vi "Main.vi"() -> ()   [LabVIEW 2015]
doc: "This template is for the Queued Message Handler design pattern.\n\nThe Event Handling Loop generates messages based on user interface actions.\n\nThe Message Handling Loop processes messages generated by the Event Handling Loop, or by other messages. The messages are string values, so new messages can be added easily to the Message Cases case structure in the Message Handling Loop. Each message cluster can also provide an optional value for Message Data, which is a variant that can be converted to whatever message-specific data is required."
uses:
  controls/UI Data.ctl
  support/Message Queue/Message Queue.lvlib
  support/User Event - Stop/User Event - Stop.lvlib
  support/Message Queue/Enqueue Message (Single).vi
  <vilib>/ErrorRing/Error Ring.xnode
  PL Model/PL Model.lvlib
  DAQ/DAQ.lvlib
  DAQ/TypeDefs/DAQ data.ctl
  support/Exit Notifiers/PLC Notifiers.lvlib
  <vilib>/Utility/error.llb/Error Cluster From Error Code.vi
  Logger/Logger.lvlib
  support/Status Logger/Status Log.ctl
panel:
  in  "Abort":bool
  in  "Stop Line":bool
  in  "Start Line":bool
  out "Status":string
  in  "Tab Control":enum32{"DAQ simulation", "DAQ control"}(tab)
  in  "Positon":dbl(slide) scale=0.0..20.0
  in  "Dispose":bool
  in  "Pump":bool
  in  "Flow [l/s]":dbl=10.0
  in  "Position (AI potentiometer)":tag
  in  "Pump (DO LED)":tag
  in  "Main switch (DI bistable switch)":tag
  in  "Dispose barrel (DI monostable switch)":tag
  in  "Exit":bool
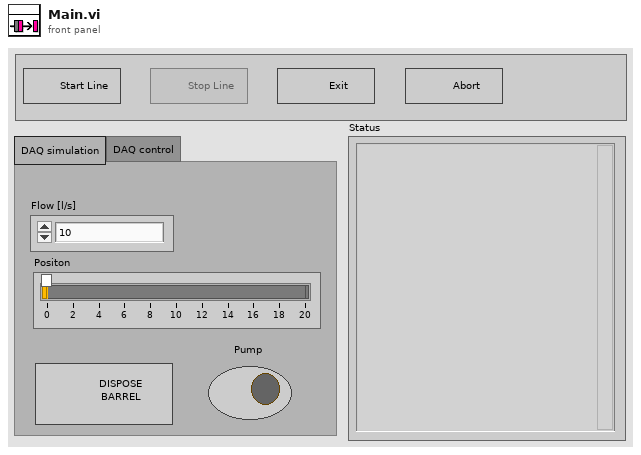
[diagram p1: front panel]
types:
  T1 = typedef "Status Log.ctl" = enum16{"Close file", "Open Status file", "Add Status", "Get file path"}
  T2 = typedef "UI Data.ctl" = cluster{"Status":string, "Start Line Ref":refnum<vi>, "Stop Line Ref":refnum<vi>, "Data Display Ref":refnum<vi>, "Exit Button Ref":refnum<vi>, "Pump Ref":refnum<vi>, "Dispose Ref":refnum<vi>, "Flow Ref":refnum<vi>, "Position Ref":refnum<vi>, "Tab Ref":refnum<vi>}
  T3 = typedef "PLC Notifiers.lvlib/PLC Notifiers.ctl" = cluster{"PL Model Exit":refnum<notifier>, "DAQ Exit":refnum<notifier>, "PLC Exit":refnum<notifier>}
  T4 = typedef "Message Queue.lvlib/All Message Queues.ctl" = cluster{"UI":refnum<queue>, "PL Model":refnum<queue>, "DAQ":refnum<queue>, "PLC":refnum<queue>, "Loger":refnum<queue>}
  T5 = typedef "DAQ.lvlib/DAQ data.ctl" = cluster{"Power switch (DI)":cluster{"Channel":tag, "Data":bool}, "Dispose barrel (DI)":cluster{"Channel":tag, "Data":bool}, "Pump status (DO)":cluster{"Channel":tag, "Data":bool}, "Barrel position (AI)":cluster{"Channel":tag, "Data":dbl}}
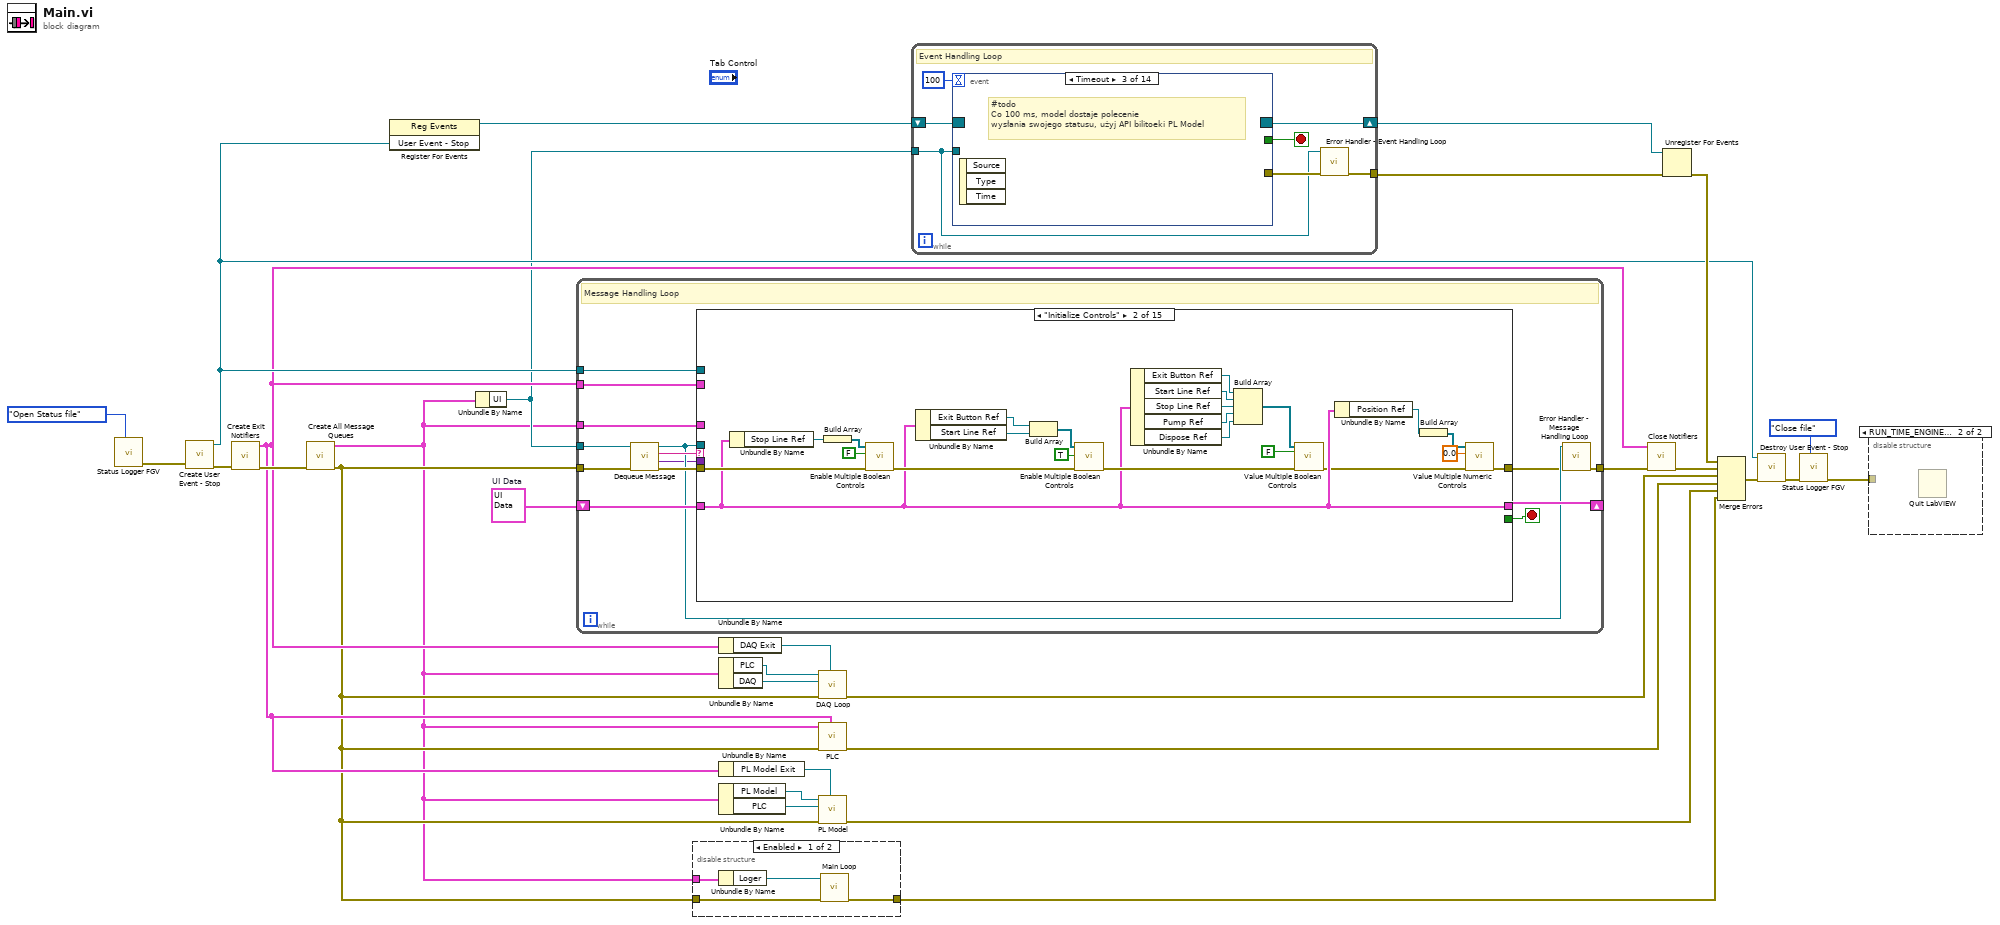
[diagram p0: block diagram]
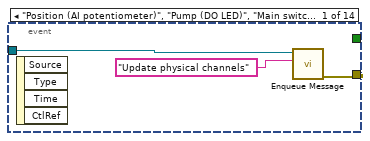
[diagram p2: hidden frame]
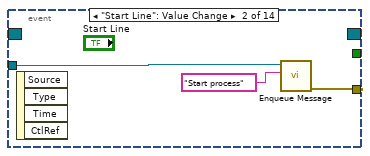
[diagram p3: hidden frame]
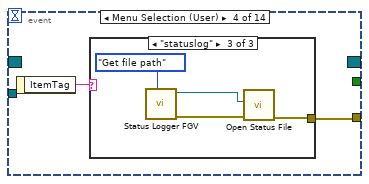
[diagram p4: hidden frame]
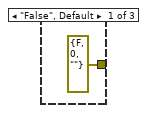
[diagram p5: hidden frame]
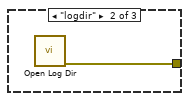
[diagram p6: hidden frame]
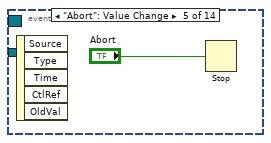
[diagram p7: hidden frame]
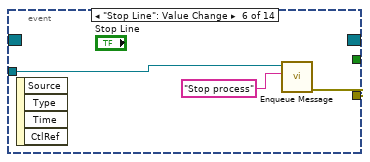
[diagram p8: hidden frame]
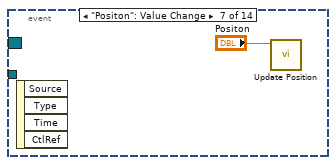
[diagram p9: hidden frame]
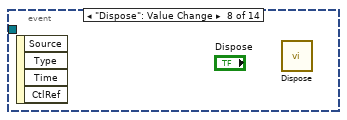
[diagram p10: hidden frame]
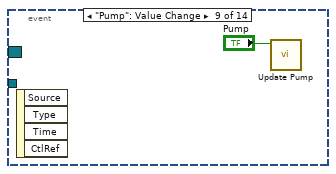
[diagram p11: hidden frame]
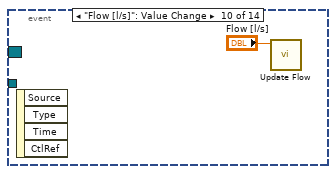
[diagram p12: hidden frame]
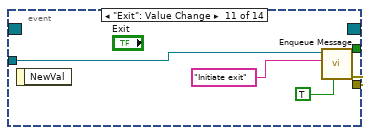
[diagram p13: hidden frame]
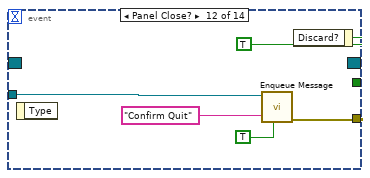
[diagram p14: hidden frame]
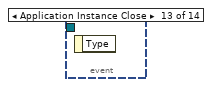
[diagram p15: hidden frame]
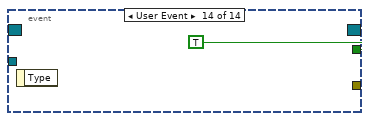
[diagram p16: hidden frame]
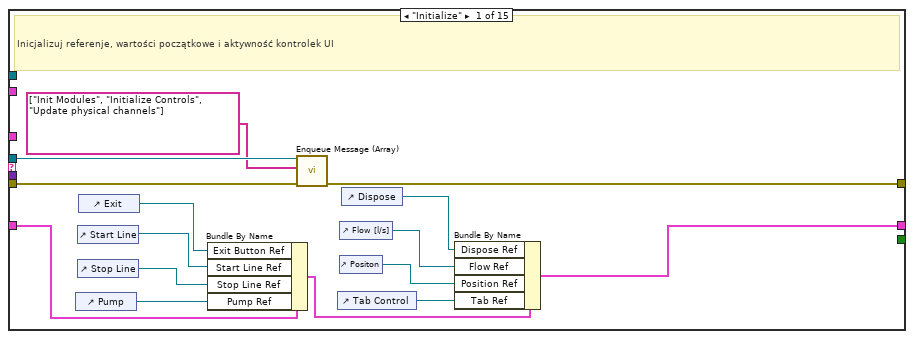
[diagram p18: hidden frame]
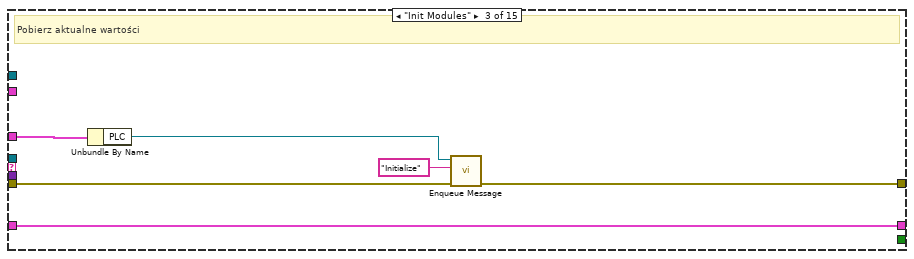
[diagram p19: hidden frame]
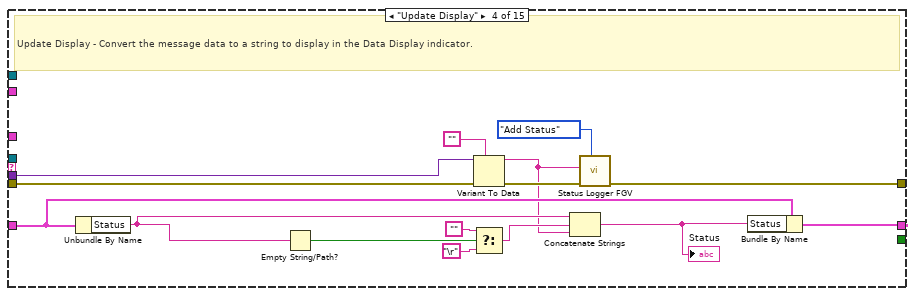
[diagram p20: hidden frame]
diagram:
  w27 = T2 {"Status"="", "Start Line Ref"=refnum, "Stop Line Ref"=refnum, "Data Display Ref"=refnum, "Exit Button Ref"=refnum, "Pump Ref"=refnum, "Dispose Ref"=refnum, "Flow Ref"=refnum, "Position Ref"=refnum, "Tab Ref"=refnum}  # UI Data
  n1 = call "Status Logger FGV.vi"("Action"=Status_Log."Open Status file") -> ("error out"=w4:errorcluster)  [unwired: 9 in, 1 out]
  n2 = call "Create User Event - Stop.vi"("error in (no error)"=w4) -> ("error out"=w19:errorcluster, "User Event - Stop"=w23:refnum<user-event>)  [unwired: 9 in]
  n3 = call "Create Exit Notifiers.vi"("error in"=w19) -> ("error out"=w18:errorcluster, "Notifiers"=w15:T3)  [unwired: 9 in]
  n4 = call "Create All Message Queues.vi"("error in (no error)"=w18) -> ("error out"=w9:errorcluster, "Message Queues out"=w7:T4)  [unwired: 9 in]
  n5 = register-events(w23) -> (reference out=w24:refnum<event-registration>)  [unwired: 2 in, 1 out]
  n6 = Unbundle By Name(w7) -> ("UI"=w8:refnum<queue>)
  n7 = while {
    tunnel: w8 -> [w37]
    shift-right: [w43] -> _
    shift-left: w27 -> [w44]
    tunnel: w23 -> [w41]
    tunnel: w9 -> [w40]
    tunnel: [w35] -> w17
    tunnel: w7 -> [w33]
    tunnel: w15 -> [w32]
    stop <- w42 stop-if-true
    # "Message Handling Loop"
    n8 = call "Dequeue Message.vi"("error in (no error)"=w40, "Message Queue"=w37) -> ("error out"=w39:errorcluster, "Message Data"=w31:variant, "Message"=w38:string, "dup Message Queue"=w36:refnum<queue>)  [unwired: 6 in]
    n9 = case "Message Cases" shown="\"Initialize Controls\"" w38 {
      selector: w38 -> [_ _ _ _ _ _ _ _ _ _ _ _ _ w226 _]
      tunnel: w36 -> [w56 _ _ _ _ _ w149 w159 _ w181 w191 w218 _ _ _]
      tunnel: w39 -> [w57 w82 w85 w103 w110 w119 w152 w163 w174 w177 w193 w209 w225 _ w238]
      tunnel: [w58 w63 w87 w89 w116 w136 w154 w161 w172 w188 w190 w207 w219 w227 w236] -> w34
      tunnel: w44 -> [w59 w65 w84 w99 w117 w125 w141 w162 w170 w189 w197 w217 w224 w228 w237]
      tunnel: [w47 w65 w84 w97 w117 w125 w141 w162 w170 w189 w197 w217 w224 w228 w237] -> w43
      tunnel: [_ _ _ _ _ _ _ _ _ _ _ TRUE _ _ _] -> w42
      tunnel: w31 -> [_ _ _ w102 _ _ _ _ w173 _ _ w210 w223 _ _]
      tunnel: w41 -> [_ _ _ _ _ _ _ _ _ _ _ w214 _ _ _]
      tunnel: w33 -> [_ _ w83 _ w106 w135 w153 _ _ w187 _ _ _ _ _]
      tunnel: w32 -> [_ _ _ _ _ _ _ _ _ _ w196 _ _ _ _]
      frame "Initialize" {
        # "Inicjalizuj referenje, wartości początkowe i aktywność kontrolek UI"
        n10 = control-ref of="Pump"() -> (w51:refnum<vi>)
        n11 = control-ref of="Start Line"() -> (w53:refnum<vi>)
        n12 = control-ref of="Stop Line"() -> (w52:refnum<vi>)
        n13 = control-ref of="Exit"() -> (w54:refnum<vi>)
        n14 = Bundle By Name(cluster=w59, "Exit Button Ref"=w54, "Start Line Ref"=w53, "Stop Line Ref"=w52, "Pump Ref"=w51) -> (w55:T2)
        n15 = call "Enqueue Message (Array).vi"("error in (no error)"=w57, "Message Array"=string[] ["Init Modules", "Initialize Controls", "Update physical channels"], "Message Queue"=w56) -> ("error out"=w58:errorcluster)  [unwired: 7 in, 1 out]
        n16 = control-ref of="Tab Control"() -> (w50:refnum<vi>)
        n17 = control-ref of="Flow [l/s]"() -> (w48:refnum<vi>)
        n18 = control-ref of="Positon"() -> (w49:refnum<vi>)
        n19 = control-ref of="Dispose"() -> (w46:refnum<vi>)
        n20 = Bundle By Name(cluster=w55, "Dispose Ref"=w46, "Flow Ref"=w48, "Position Ref"=w49, "Tab Ref"=w50) -> (w47:T2)
      }
      frame "Initialize Controls" {
        n21 = Unbundle By Name(w65) -> ("Stop Line Ref"=w80:refnum<vi>)
        n22 = Build Array(w80) -> (w79:refnum<vi>[])
        n23 = call "Enable Multiple Boolean Controls.vi"("error in (no error)"=w82, "Enabled"=FALSE, "References"=w79) -> ("error out"=w76:errorcluster)  [unwired: 8 in]
        n24 = Unbundle By Name(w65) -> ("Exit Button Ref"=w78:refnum<vi>, "Start Line Ref"=w77:refnum<vi>)
        n25 = Build Array(w78, w77) -> (w75:refnum<vi>[])
        n26 = call "Enable Multiple Boolean Controls.vi"("error in (no error)"=w76, "Enabled"=TRUE, "References"=w75) -> ("error out"=w68:errorcluster)  [unwired: 8 in]
        n27 = Unbundle By Name(w65) -> ("Exit Button Ref"=w73:refnum<vi>, "Start Line Ref"=w72:refnum<vi>, "Stop Line Ref"=w71:refnum<vi>, "Pump Ref"=w70:refnum<vi>, "Dispose Ref"=w69:refnum<vi>)
        n28 = Build Array(w73, w72, w71, w70, w69) -> (w66:refnum<vi>[])
        n29 = call "Value Multiple Boolean Controls.vi"("error in (no error)"=w68, "Enabled"=FALSE, "References"=w66) -> ("error out"=w64:errorcluster)  [unwired: 8 in]
        n30 = Unbundle By Name(w65) -> ("Position Ref"=w62:refnum<vi>)
        n31 = Build Array(w62) -> (w61:refnum<vi>[])
        n32 = call "Value Multiple Numeric Controls.vi"("error in (no error)"=w64, "Value"=0.0, "References"=w61) -> ("error out"=w63:errorcluster)  [unwired: 8 in]
      }
      frame "Init Modules" {
        # "Pobierz aktualne wartości"
        n33 = Unbundle By Name(w83) -> ("PLC"=w86:refnum<queue>)
        n34 = call-poly "Enqueue Message.vi"("error in (no error)"=w85, "Message"="Initialize", "Message Queue"=w86) -> ("error out"=w87:errorcluster)  [unwired: 7 in, 1 out]
      }
      frame "Update Display" {
        # "Update Display - Convert the message data to a string to display in the Data Display indicator."
        n35 = Unbundle By Name(w99) -> ("Status"=w96:string)
        n36 = Empty String/Path?(string/path=w96) -> (empty?=w95:bool)
        n37 = Variant To Data(error in=w103, type="", Variant=w102) -> (data=w91:string, error out=w100:errorcluster)
        n38 = Select(t="", s=w95, f="\r") -> (s? t:f=w92:string)
        n39 = Concatenate Strings(w96, w92, w91) -> (w98:string)
        "Status" <- w98
        n40 = call "Status Logger FGV.vi"("Action"=Status_Log."Add Status", "error in (no error)"=w100, "Status"=w91) -> ("error out"=w89:errorcluster)  [unwired: 7 in, 1 out]
        n41 = Bundle By Name(cluster=w99, "Status"=w98) -> (w97:T2)
      }
      frame "Update physical channels" {
        # "Duplicate this frame when creating new messages.  Change this comment in the duplicated frame to describe this message."
        n42 = Bundle By Name(cluster=T5 {"Power switch (DI)"={"Channel"="", "Data"=FALSE}, "Dispose barrel (DI)"={"Channel"="", "Data"=FALSE}, "Pump status (DO)"={"Channel"="", "Data"=FALSE}, "Barrel position (AI)"={"Channel"="", "Data"=0.0}} ("DAQ data"), "Power switch (DI).Channel"="Main switch (DI bistable switch)", "Pump status (DO).Channel"="Pump (DO LED)", "Barrel position (AI).Channel"="Position (AI potentiometer)", "Dispose barrel (DI).Channel"="Dispose barrel (DI monostable switch)") -> (w108:T5)
        n43 = Unbundle By Name(w106) -> ("PLC"=w105:refnum<queue>)
        n44 = To Variant(anything=w108) -> (Variant=w107:variant)
        n45 = call-poly "Enqueue Message.vi"("error in (no error)"=w110, "Message Data"=w107, "Message"="Update channels", "Message Queue"=w105) -> ("error out"=w109:errorcluster)  [unwired: 6 in, 1 out]
        n46 = Merge Errors(w109) -> (w116:errorcluster)
      }
      frame "Start process" {
        # "Duplicate this frame when creating new messages.  Change this comment in the duplicated frame to describe this message."
        n47 = Unbundle By Name(w125) -> ("Start Line Ref"=w128:refnum<vi>)
        n48 = Unbundle By Name(w125) -> ("Stop Line Ref"=w124:refnum<vi>)
        n49 = Unbundle By Name(w135) -> ("UI"=w121:refnum<queue>, "PLC"=w134:refnum<queue>, "Loger"=w118:refnum<queue>)
        n50 = call "Open Log.vi"("error in (no error)"=w119, "Message Queue"=w118) -> ("error out"=w120:errorcluster)  [unwired: 9 in]
        n51 = Build Array(w128) -> (w127:refnum<vi>[])
        n52 = Build Array(w124) -> (w123:refnum<vi>[])
        n53 = call-poly "Enqueue Message.vi"("error in (no error)"=w120, "Message"="Start", "Message Queue"=w134) -> ("error out"=w132:errorcluster)  [unwired: 7 in, 1 out]
        n54 = call "Enable Multiple Boolean Controls.vi"("Enabled"=FALSE, "References"=w127) -> ()  [unwired: 9 in, 1 out]
        n55 = call "Enable Multiple Boolean Controls.vi"("Enabled"=TRUE, "References"=w123) -> ()  [unwired: 9 in, 1 out]
        n56 = call-poly "Enqueue Message.vi"("error in (no error)"=w132, "Message Data"="Starting production line..." ("Message"), "Message"="Update Display", "Message Queue"=w121) -> ("error out"=w131:errorcluster)  [unwired: 6 in, 1 out]
        n57 = Merge Errors(w131) -> (w136:errorcluster)
      }
      frame "Stop process" {
        # "Duplicate this frame when creating new messages.  Change this comment in the duplicated frame to describe this message."
        n58 = Unbundle By Name(w141) -> ("Start Line Ref"=w144:refnum<vi>)
        n59 = Unbundle By Name(w141) -> ("Stop Line Ref"=w140:refnum<vi>)
        n60 = Unbundle By Name(w153) -> ("PLC"=w151:refnum<queue>)
        n61 = Build Array(w144) -> (w143:refnum<vi>[])
        n62 = Build Array(w140) -> (w139:refnum<vi>[])
        n63 = call-poly "Enqueue Message.vi"("error in (no error)"=w152, "Message"="Stop", "Message Queue"=w151) -> ("error out"=w148:errorcluster)  [unwired: 7 in, 1 out]
        n64 = To Variant(anything="Stopping production line..." ("Message")) -> (Variant=w137:variant)
        n65 = call "Enable Multiple Boolean Controls.vi"("Enabled"=TRUE, "References"=w143) -> ()  [unwired: 9 in, 1 out]
        n66 = call "Enable Multiple Boolean Controls.vi"("Enabled"=FALSE, "References"=w139) -> ()  [unwired: 9 in, 1 out]
        n67 = call-poly "Enqueue Message.vi"("error in (no error)"=w148, "Message Data"=w137, "Message"="Update Display", "Message Queue"=w149) -> ("error out"=w147:errorcluster)  [unwired: 6 in, 1 out]
        n68 = Merge Errors(w147) -> (w154:errorcluster)
      }
      frame "Confirm Quit" {
        # "Confirm Quit - Message that can confirm whether or not the user wants to exit the application."
        n69 = Two Button Dialog(message="Are you sure?", 1:"Continue" ("F button name (\"Cancel\")"), 2:"Quit" ("T button name (\"OK\")")) -> (T button?=w155:bool)
        n70 = case shown="True" w155 {
          tunnel: w163 -> [w164 w169]
          tunnel: [w164 w168] -> w160
          tunnel: w159 -> [_ w167]
          frame False {
          }
          frame True {
            n71 = call-poly "Enqueue Message.vi"("Priority Message? (F)"=TRUE, "error in (no error)"=w169, "Message"="Initiate exit", "Message Queue"=w167) -> ("error out"=w168:errorcluster)  [unwired: 6 in, 1 out]
          }
        }
        n72 = Merge Errors(w160) -> (w161:errorcluster)
      }
      frame "Update PL Status" {
        n73 = Variant To Data(error in=w174, type="", Variant=w173) -> (error out=w172:errorcluster)  [unwired: 1 out]
      }
      frame "Initiate exit" {
        # "Exit - Exit the application."
        n74 = Unbundle By Name(w187) -> ("PLC"=w186:refnum<queue>, "Loger"=w175:refnum<queue>)
        n75 = call "Exit.vi"("error in (no error)"=w177, "Message Queue"=w175) -> ("error out"=w176:errorcluster)  [unwired: 9 in]
        n76 = call-poly "Enqueue Message.vi"("Priority Message? (F)"=TRUE, "error in (no error)"=w176, "Message"="Exit PLC", "Message Queue"=w186) -> ("error out"=w179:errorcluster)  [unwired: 6 in, 1 out]
        n77 = Flush Queue(queue=w181, error in (no error)=w179) -> (queue out=w180:refnum<queue>, error out=w178:errorcluster)  [unwired: 1 out]
        n78 = call-poly "Enqueue Message.vi"("error in (no error)"=w178, "Message"="Wait on PLC exit", "Message Queue"=w180) -> ("error out"=w184:errorcluster)  [unwired: 7 in, 1 out]
        n79 = Merge Errors(w184) -> (w188:errorcluster)
      }
      frame "Wait on PLC exit" {
        # "Exit - Exit the application."
        n80 = Unbundle By Name(w196) -> ("PLC Exit"=w195:refnum<notifier>)
        n81 = Wait on Notification(notifier=w195, timeout in ms (-1)=10, error in (no error)=w193) -> (timed out?=w192:bool)  [unwired: 1 in, 3 out]
        n82 = case shown="True" w192 {
          tunnel: [w200 w204] -> w190
          tunnel: w193 -> [w199 w203]
          tunnel: w191 -> [w198 w202]
          frame True {
            n83 = call-poly "Enqueue Message.vi"("error in (no error)"=w199, "Message"="Wait on PLC exit", "Message Queue"=w198) -> ("error out"=w200:errorcluster)  [unwired: 7 in, 1 out]
          }
          frame False {
            n84 = call-poly "Enqueue Message.vi"("error in (no error)"=w203, "Message"="Exit", "Message Queue"=w202) -> ("error out"=w204:errorcluster)  [unwired: 7 in, 1 out]
          }
        }
      }
      frame "Exit" {
        # "Release the message queue reference"
        # "Exit - Exit the application."
        n85 = Variant To Data(type=errorcluster {"status"=FALSE, "code"=0, "source"=""} ("error constant"), Variant=w210) -> (data=w211:errorcluster)  [unwired: 1 in, 1 out]
        n86 = call <vilib>:"Simple Error Handler.vi"("error in (no error)"=w211) -> ()  [unwired: 4 in, 5 out]
        n87 = Release Queue(queue=w218, force destroy? (F)=TRUE, error in (no error)=w209) -> (error out=w215:errorcluster)  [unwired: 2 out]
        n88 = call "Fire User Event - Stop.vi"("User Event - Stop"=w214) -> ("error out"=w213:errorcluster)  [unwired: 10 in]
        n89 = Merge Errors(w213, w215) -> (w208:errorcluster)
        n90 = call "Exit.vi"("error in (no error)"=w208) -> ("error out"=w207:errorcluster)  [unwired: 10 in]
      }
      frame "Error" {
        # "Error - Display an error dialog. This message is sent by the \"Error Handler\" VIs at the end of other loops in this application."
        n91 = Variant To Data(error in=w225, type=errorcluster {"status"=FALSE, "code"=0, "source"=""} ("error constant"), Variant=w223) -> (data=w221:errorcluster, error out=w220:errorcluster)
        n92 = call <vilib>:"Simple Error Handler.vi"("error in (no error)"=w221) -> ()  [unwired: 4 in, 5 out]
        n93 = Merge Errors(w220) -> (w219:errorcluster)
      }
      frame Default {
        # "'Default' case only runs if there is a message that isn't defined in any of the other cases.  Output a programming error."
        n94 = xnode "Error Ring"("parameter 0"=w226) -> ("error out"=w227:errorcluster)
      }
      frame "---Copy This Frame---" {
        # "Duplicate this frame when creating new messages.  Change this comment in the duplicated frame to describe this message."
        n95 = Merge Errors(w238) -> (w236:errorcluster)
      }
    }
    n96 = call "Error Handler - Message Handling Loop.vi"("error in (no error)"=w34, "Message Queue"=w36) -> ("dup error in"=w35:errorcluster)  [unwired: 8 in, 1 out]
  }
  n97 = disable-structure shown="Enabled" {
    disable-tunnel: [w242 _] -> w10
    disable-tunnel: w9 -> [w241 _]
    disable-tunnel: w7 -> [w240 _]
    frame Enabled {
      n98 = Unbundle By Name(w240) -> ("Loger"=w239:refnum<queue>)
      n99 = call "Main Loop.vi"("error in (no error)"=w241, "Queue in"=w239) -> ("error out"=w242:errorcluster)  [unwired: 9 in]
    }
    frame Disabled {
    }
  }
  n100 = Unbundle By Name(w15) -> ("DAQ Exit"=w16:refnum<notifier>)
  n101 = Unbundle By Name(w7) -> ("PLC"=w21:refnum<queue>, "DAQ"=w20:refnum<queue>)
  n102 = Unbundle By Name(w15) -> ("PL Model Exit"=w14:refnum<notifier>)
  n103 = Unbundle By Name(w7) -> ("PL Model"=w22:refnum<queue>, "PLC"=w11:refnum<queue>)
  n104 = call "DAQ Loop.vi"("DAQ Exit"=w16, "error in"=w9, "DAQ Queue"=w20, "PLC Queue"=w21) -> ("error out"=w5:errorcluster)  [unwired: 7 in]
  n105 = call "PLC.vi"("Notifiers"=w15, "error in"=w9, "Message Queues"=w7) -> ("error out"=w6:errorcluster)  [unwired: 8 in]
  n106 = call "PL Model.vi"("PL Model Exit"=w14, "error in (no error)"=w9, "Controller queue"=w11, "Message Queue In"=w22) -> ("error out"=w12:errorcluster)  [unwired: 7 in]
  n107 = while {
    tunnel: w8 -> [w243]
    shift-right: [w248] -> w28
    shift-left: w24 -> [w249]
    tunnel: [w245] -> w25
    stop <- w246 stop-if-true
    # "Event Handling Loop"
    n108 = event shown="[2] Timeout" {
      selector: w249 -> [_ _ _ _ _ _ _ _ _ _ _ _ _ _]
      dyn-events: [_ _ _ _ _ _ _ _ _ _ _ _ _ _] -> w248
      timeout: 100 -> [_ _ _ _ _ _ _ _ _ _ _ _ _ _]
      tunnel: [_ _ _ _ _ _ _ _ _ _ _ _ _ TRUE ("Discard?")] -> w246
      tunnel: w243 -> [w252 w255 _ _ _ w267 _ _ _ _ w274 w278 _ _]
      tunnel: [w251 w254 _ w256 _ w266 _ _ _ _ w273 w277 _ _] -> w247
      event "Position (AI potentiometer)", "Pump (DO LED)", "Main switch (DI bistable switch)", "Dispose barrel (DI monostable switch)": Value Change {
        n109 = event-data() -> ()  [unwired: 1 in, 4 out]
        n110 = call-poly "Enqueue Message.vi"("Message"="Update physical channels", "Message Queue"=w252) -> ("error out"=w251:errorcluster)  [unwired: 8 in, 1 out]
      }
      event "Start Line": Value Change {
        n111 = event-data() -> ()  [unwired: 1 in, 4 out]
        n112 = call-poly "Enqueue Message.vi"("Message"="Start process", "Message Queue"=w255) -> ("error out"=w254:errorcluster)  [unwired: 8 in, 1 out]
      }
      event Timeout {
        # "#todo \nCo 100 ms, model dostaje polecenie \nwysłania swojego statusu, użyj API bilitoeki PL Model"
        n113 = event-data() -> ()  [unwired: 1 in, 3 out]
      }
      event Menu Selection (User) {
        n114 = event-data() -> ("ItemTag"=w257:string)  [unwired: 1 in]
        n115 = case shown="\"statuslog\"" w257 {
          tunnel: [errorcluster {"status"=FALSE, "code"=0, "source"=""} ("error out") w259 w262] -> w256
          frame "False", Default {
          }
          frame "logdir" {
            n116 = call "Open Log Dir.vi"() -> ("error out"=w259:errorcluster)  [unwired: 11 in]
          }
          frame "statuslog" {
            n117 = call "Status Logger FGV.vi"("Action"=Status_Log."Get file path") -> ("error out"=w261:errorcluster, "Staus Log Path"=w260:path)  [unwired: 9 in]
            n118 = call "Open Status File.vi"("error in (no error)"=w261, "path"=w260) -> ("error out"=w262:errorcluster)  [unwired: 9 in]
          }
        }
      }
      event "Abort": Value Change {
        n119 = event-data() -> ()  [unwired: 1 in, 5 out]
        n120 = Stop(stop? (T)="Abort") -> ()
      }
      event "Stop Line": Value Change {
        n121 = event-data() -> ()  [unwired: 1 in, 4 out]
        n122 = call-poly "Enqueue Message.vi"("Message"="Stop process", "Message Queue"=w267) -> ("error out"=w266:errorcluster)  [unwired: 8 in, 1 out]
      }
      event "Positon": Value Change {
        n123 = event-data() -> ()  [unwired: 1 in, 4 out]
        n124 = call "Update Position.vi"("Position"="Positon") -> ()  [unwired: 10 in, 1 out]
      }
      event "Dispose": Value Change {
        n125 = event-data() -> ()  [unwired: 1 in, 4 out]
        n126 = call "Dispose.vi"() -> ()  [unwired: 11 in, 1 out]
      }
      event "Pump": Value Change {
        n127 = event-data() -> ()  [unwired: 1 in, 4 out]
        n128 = call "Update Pump.vi"("Pump State"="Pump") -> ()  [unwired: 10 in, 1 out]
      }
      event "Flow [l/s]": Value Change {
        n129 = event-data() -> ()  [unwired: 1 in, 4 out]
        n130 = call "Update Flow.vi"("Flow"="Flow [l/s]") -> ()  [unwired: 10 in, 1 out]
      }
      event "Exit": Value Change {
        n131 = event-data() -> ()  [unwired: 1 in, 1 out]
        n132 = call-poly "Enqueue Message.vi"("Priority Message? (F)"=TRUE, "Message"="Initiate exit", "Message Queue"=w274) -> ("error out"=w273:errorcluster)  [unwired: 7 in, 1 out]
      }
      event Panel Close? {
        n133 = event-data() -> ()  [unwired: 1 in, 1 out]
        n134 = call-poly "Enqueue Message.vi"("Priority Message? (F)"=TRUE, "Message"="Confirm Quit", "Message Queue"=w278) -> ("error out"=w277:errorcluster)  [unwired: 7 in, 1 out]
        n135 = event-data("Discard?"=TRUE) -> ()  [unwired: 1 in, 1 out]
      }
      event Application Instance Close {
        n136 = event-data() -> ()  [unwired: 1 in, 1 out]
      }
      event User Event {
        n137 = event-data() -> ()  [unwired: 1 in, 1 out]
      }
    }
    n138 = call "Error Handler - Event Handling Loop.vi"("error in (no error)"=w247, "Message Queue"=w243) -> ("dup error in"=w245:errorcluster)  [unwired: 8 in, 1 out]
  }
  n139 = call "Close Notifiers.vi"("error in"=w17, "Notifiers"=w15) -> ("error out"=w13:errorcluster)  [unwired: 9 in]
  n140 = Unregister For Events(event registration refnum=w28, error in=w25) -> (error out=w29:errorcluster)
  n141 = Merge Errors(w29, w13, w5, w6, w12, w10) -> (w30:errorcluster)
  n142 = call "Destroy User Event - Stop.vi"("error in (no error)"=w30, "User Event - Stop"=w23) -> ("error out"=w26:errorcluster)  [unwired: 9 in]
  n143 = call "Status Logger FGV.vi"("Action"=Status_Log."Close file", "error in (no error)"=w26) -> ("error out"=w2:errorcluster)  [unwired: 8 in, 1 out]
  n144 = disable-structure shown="RUN_TIME_ENGINE==True" {
    disable-tunnel: w2 -> [_ _]
    frame condition #0 (active) {
    }
    frame condition #1 {
      n145 = Quit LabVIEW() -> ()  [unwired: 1 in]
    }
  }
